vi "Check for Message.vi"(9 "error in":errorcluster, 11 "module reference":T1) -> (1 "error out":errorcluster, 3 "new element available":bool)   [LabVIEW 2017, in "myPAM.lvlib"]
uses:
  myPAM.lvlib
  Private TypeDefs/Module Reference.ctl
  Global TypeDefs/Registered Modules.ctl
  Private TypeDefs/Module Queues.ctl
  Private TypeDefs/Message Queue Element.ctl
  Public TypeDefs/Messages.ctl
  Private TypeDefs/Module Notifiers.ctl
  Public TypeDefs/Current Position Data.ctl
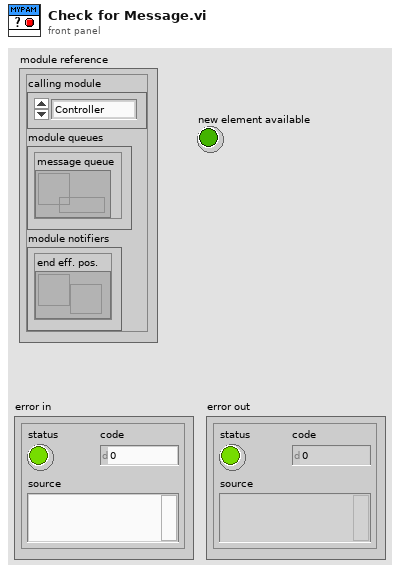
[diagram p1: front panel]
types:
  T1 = typedef "myPAM.lvlib/Module Reference.ctl" = cluster{"calling module":T2, "module queues":T3, "module notifiers":T4}
  T2 = typedef "Registered Modules.ctl" = enum16{"Controller", "DAQ", "Error Handler", "Game", "myPAM", "WinHost", "Logger"}
  T3 = typedef "myPAM.lvlib/Module Queues.ctl" = cluster{"message queue":refnum<queue>}
  T4 = typedef "myPAM.lvlib/Module Notifiers.ctl" = cluster{"end eff. pos.":refnum<notifier>}
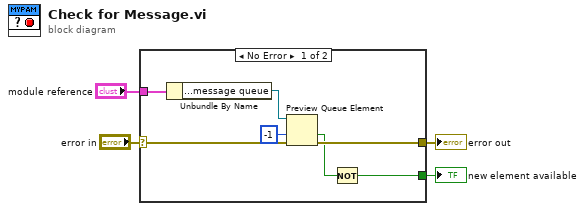
[diagram p0: block diagram]
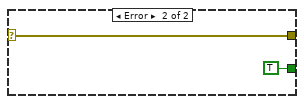
[diagram p2: hidden frame]
diagram:
  n1 = case shown="No Error" "error in" {
    selector: "error in" -> [w11 w13]
    tunnel: "module reference" -> [w10 _]
    tunnel: [w8 w13] -> w2
    tunnel: [w6 TRUE] -> w1
    frame No Error {
      n2 = Unbundle By Name(w10) -> ("module queues.message queue"=w9:refnum<queue>)
      n3 = Preview Queue Element(queue=w9, timeout in ms (-1)=-1, error in (no error)=w11) -> (timed out?=w7:bool, error out=w8:errorcluster)  [unwired: 2 out]
      n4 = Not(x=w7) -> (.not. x?=w6:bool)
    }
    frame Error {
    }
  }
  "error out" <- w2
  "new element available" <- w1
